vi "添加设备.vi"(8 "error in (no error)":errorcluster, 10 "设备名称":string, 11 "数据库连接引用 i":T1) -> (0 "error out":errorcluster, 3 "数据库连接引用 o":T1)   [LabVIEW 2017]
uses:
  <vilib>/addons/database/Connection.llb/Conn ObjectReference.ctl
  <vilib>/addons/database/Connection.llb/Conn Execute.vi
  <vilib>/addons/database/NI_Database_API.lvlib
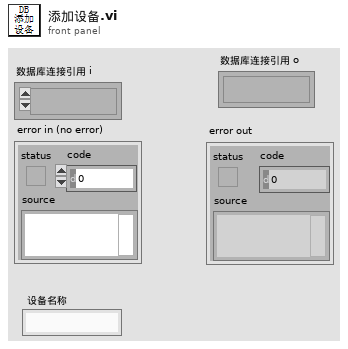
[diagram p1: front panel]
types:
  T1 = typedef "NI_Database_API.lvlib/Conn ObjectReference.ctl" = refnum<k1>
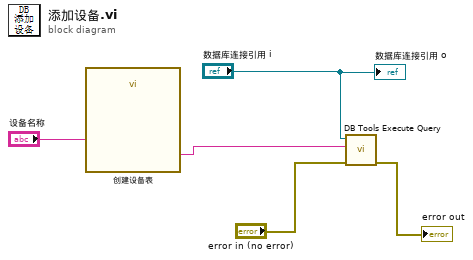
[diagram p0: block diagram]
diagram:
  n1 = call "创建设备表"("设备名称"="设备名称") -> ("Result"=w3:string)  [unwired: 13 in, 1 out]
  n2 = call-poly <vilib>:"DB Tools Execute Query.vi"("error in (no error)"="error in (no error)", "SQL query"=w3, "connection reference"="数据库连接引用 i") -> ("error out"=→"error out":errorcluster)  [unwired: 5 in, 1 out]
  "数据库连接引用 o" <- "数据库连接引用 i"
